vi "Set New Direction.vi"(10 "New Direction":T1, 11 "Target Direction in":T2) -> (3 "Target Direction out":T2)   [LabVIEW 2020, in "AntFarm_MB.lvclass"]
uses:
  AntFarm_MB.lvclass
  Type Defs/Direction Enum.ctl
  TypeDefs/ENUM_New Direction Select.ctl
  Type Defs/SB Type Defs.lvlib
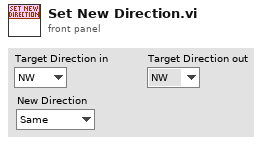
[diagram p1: front panel]
types:
  T1 = typedef "ENUM_New Direction Select.ctl" = enum16{"Same", "CCW 45", "CW 45", "CCW 90", "CW 90", "CCW 135", "CW 135", "Opposite"}
  T2 = typedef "SB Type Defs.lvlib/Direction Enum.ctl" = enum16{"NW", "N", "NE", "E", "SE", "S", "SW", "W"}
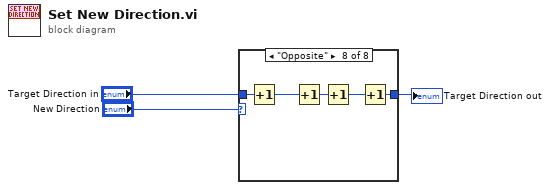
[diagram p0: block diagram]
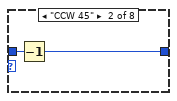
[diagram p3: hidden frame]
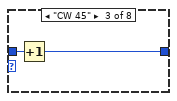
[diagram p4: hidden frame]
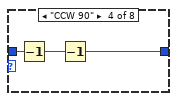
[diagram p5: hidden frame]
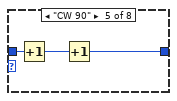
[diagram p6: hidden frame]
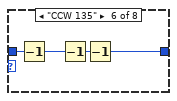
[diagram p7: hidden frame]
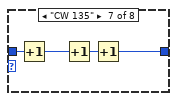
[diagram p8: hidden frame]
diagram:
  n1 = case shown="\"Opposite\"" "New Direction" {
    tunnel: "Target Direction in" -> [w4 w6 w8 w11 w14 w18 w22 w27]
    tunnel: [w4 w5 w7 w9 w12 w15 w19 w23] -> w1
    frame "Same" {
    }
    frame "CCW 45" {
      n2 = Decrement(x=w6) -> (x-1=w5:T2)
    }
    frame "CW 45" {
      n3 = Increment(x=w8) -> (x+1=w7:T2)
    }
    frame "CCW 90" {
      n4 = Decrement(x=w11) -> (x-1=w10:T2)
      n5 = Decrement(x=w10) -> (x-1=w9:T2)
    }
    frame "CW 90" {
      n6 = Increment(x=w14) -> (x+1=w13:T2)
      n7 = Increment(x=w13) -> (x+1=w12:T2)
    }
    frame "CCW 135" {
      n8 = Decrement(x=w18) -> (x-1=w17:T2)
      n9 = Decrement(x=w17) -> (x-1=w16:T2)
      n10 = Decrement(x=w16) -> (x-1=w15:T2)
    }
    frame "CW 135" {
      n11 = Increment(x=w22) -> (x+1=w21:T2)
      n12 = Increment(x=w21) -> (x+1=w20:T2)
      n13 = Increment(x=w20) -> (x+1=w19:T2)
    }
    frame "Opposite" {
      n14 = Increment(x=w27) -> (x+1=w26:T2)
      n15 = Increment(x=w26) -> (x+1=w25:T2)
      n16 = Increment(x=w25) -> (x+1=w24:T2)
      n17 = Increment(x=w24) -> (x+1=w23:T2)
    }
  }
  "Target Direction out" <- w1
